vi "GetWidthAndHeight.vi"(0 "camera cluster":T3) -> (1 "Width":u32, 2 "Height":u32)   [LabVIEW 2015]
uses:
  <vilib>/vision/Avi1.llb/AviRefnum.ctl
  <vilib>/userdefined/High Color/IMAQdx.ctl
  <resource>/objmgr/imaqdx.rc
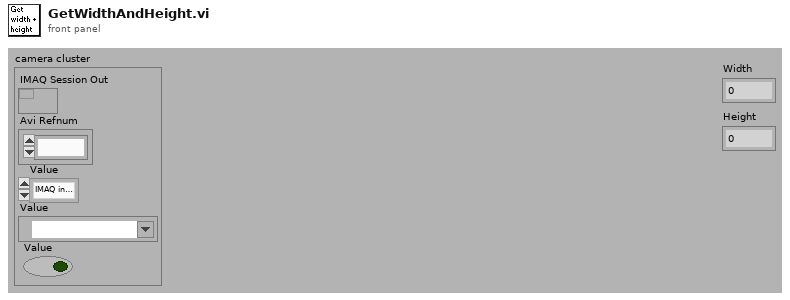
[diagram p1: front panel]
types:
  T1 = typedef "AviRefnum.ctl" = refnum<k1>
  T2 = typedef "IMAQdx.ctl" = refnum<k21>
  T3 = cluster{"IMAQ Session Out":refnum<k11>, "Avi Refnum":T1, "Value":enum32{"IMAQ interface", "IMAQdx interface", "AVI file"}, "Value":T2, "Value":bool}
  T4 = enum32{"IMAQ interface", "IMAQdx interface", "AVI file"}
  T5 = cluster{"width":u32, "height":u32, "framesPerSecond":u32, "compressionFilter":string, "hasData":bool}
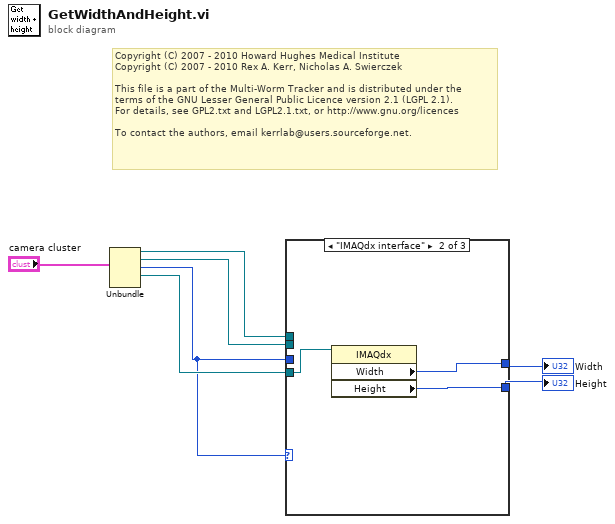
[diagram p0: block diagram]
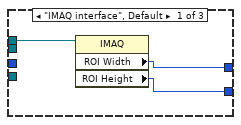
[diagram p2: hidden frame]
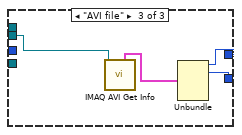
[diagram p3: hidden frame]
diagram:
  # "Copyright (C) 2007 - 2010 Howard Hughes Medical Institute\nCopyright (C) 2007 - 2010 Rex A. Kerr, Nicholas A. Swierczek\n \nThis file is a part of the Multi-Worm Tracker and is distributed under the\nterms of the GNU Lesser General Public Licence version 2.1 (LGPL 2.1).\nFor details, see GPL2.txt and LGPL2.1.txt, or http://www.gnu.org/licences\n \nTo contact the authors, email kerrlab@users.sourceforge.net."
  n1 = Unbundle("camera cluster") -> ("IMAQ Session Out"=w7:refnum<k11>, "Avi Refnum"=w3:T1, "Value"=w2:T4, "Value"=w4:T2)  [unwired: 1 out]
  n2 = case shown="\"IMAQdx interface\"" w2 {
    tunnel: w4 -> [_ w11 _]
    tunnel: w7 -> [w10 _ _]
    tunnel: [w9 w13 w16] -> w6
    tunnel: [w8 w12 w15] -> w5
    tunnel: w2 -> [_ _ _]
    tunnel: w3 -> [_ _ w14]
    frame "IMAQ interface", Default {
      n3 = property class="IMAQ"(reference=w10) -> ("ROI Width"=w9:u32, "ROI Height"=w8:u32)  [unwired: 1 in, 2 out]
    }
    frame "IMAQdx interface" {
      n4 = property class="IMAQdx"(reference=w11) -> ("Width"=w13:u32, "Height"=w12:u32)  [unwired: 1 in, 2 out]
    }
    frame "AVI file" {
      n5 = call "IMAQ AVI Get Info"("Avi Refnum"=w14) -> ("Frame Data"=w17:T5)  [unwired: 6 in, 4 out]
      n6 = Unbundle(w17) -> ("width"=w16:u32, "height"=w15:u32)  [unwired: 3 out]
    }
  }
  "Width" <- w6
  "Height" <- w5
